vi "4.9.1.vi"() -> ()   [LabVIEW 2018]
panel:
  out "c2":dbl
  out "c":dbl
  in  "b":dbl
  in  "a":dbl
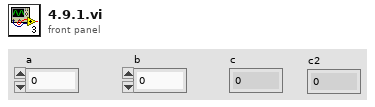
[diagram p1: front panel]
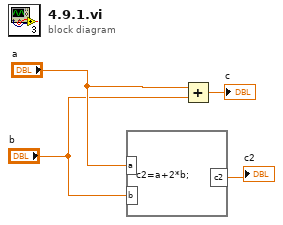
[diagram p0: block diagram]
diagram:
  n1 = formula code="c2=a+2*b;"("a"="a", "b"="b") -> ("c2"=→"c2":dbl)
  n2 = Add(x="a", y="b") -> (x+y=→"c":dbl)
